vi "ClientNetworkInterfaceGlobalVariables.vi"() -> ()   [LabVIEW 2025]
panel:
  out "Send Data Queue":refnum<queue>
  out "Receive Data Queue":refnum<queue>
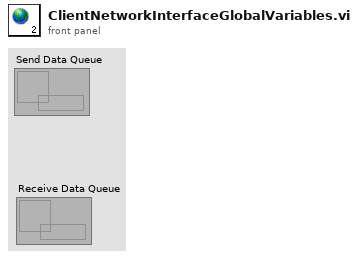
[diagram p1: front panel]
diagram:
